vi "xbee_write.vi"(8 "error in":errorcluster, 9 "value":string="+++", 10 "command":string="+++", 11 "com in":refnum<visa-resource-name>) -> (0 "error out":errorcluster, 3 "com out":refnum<visa-resource-name>)   [LabVIEW 2012]
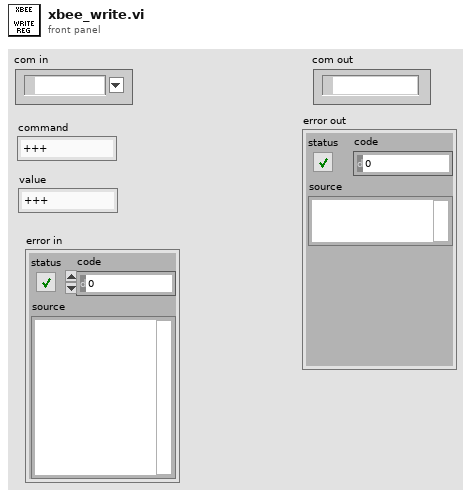
[diagram p1: front panel]
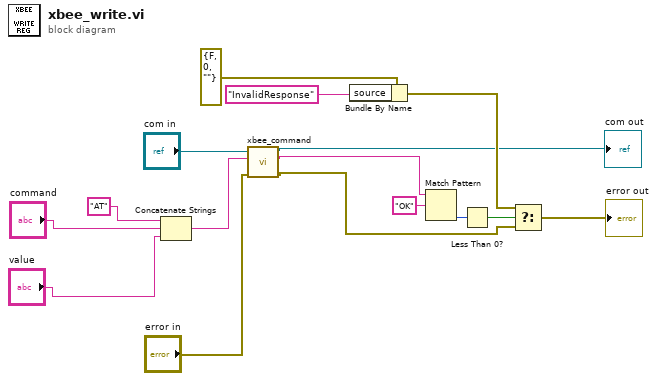
[diagram p0: block diagram]
diagram:
  n1 = Concatenate Strings("AT", "command", "value") -> (w4:string)
  n2 = call "xbee_command.vi"("error in (no error)"="error in", "command"=w4, "COM in"="com in") -> ("error out"=w7:errorcluster, "read buffer"=w8:string, "COM out"=→"com out":refnum<visa-resource-name>)  [unwired: 6 in]
  n3 = Bundle By Name(cluster=errorcluster {"status"=FALSE, "code"=0, "source"=""} ("error constant"), "source"="InvalidResponse") -> (w9:errorcluster)
  n4 = Match Pattern(string=w8, regular expression="OK") -> (offset past match=w13:i32)  [unwired: 1 in, 3 out]
  n5 = Less Than 0?(x=w13) -> (x < 0?=w14:bool)
  n6 = Select(t=w9, s=w14, f=w7) -> (s? t:f=→"error out":errorcluster)
